vi "Append Report Text (str).vi"(0 "report in":refnum<class "NI_report.lvclass">, 1 "MS Office parameters":T1, 2 "format string (%.3f)":string="%.3f", 7 "text":string, 9 "append on new line? (F)":bool, 11 "error in (no error)":errorcluster) -> (4 "report out":refnum<class "NI_report.lvclass">, 8 "start out (Word)":i32, 10 "end out (Word)":i32, 15 "error out":errorcluster)   [LabVIEW 2020, in "NI_report.lvclass"]
doc: "Appends text to the selected report."
uses:
  <vilib>/Utility/NIReport.llb/NI_report.lvclass
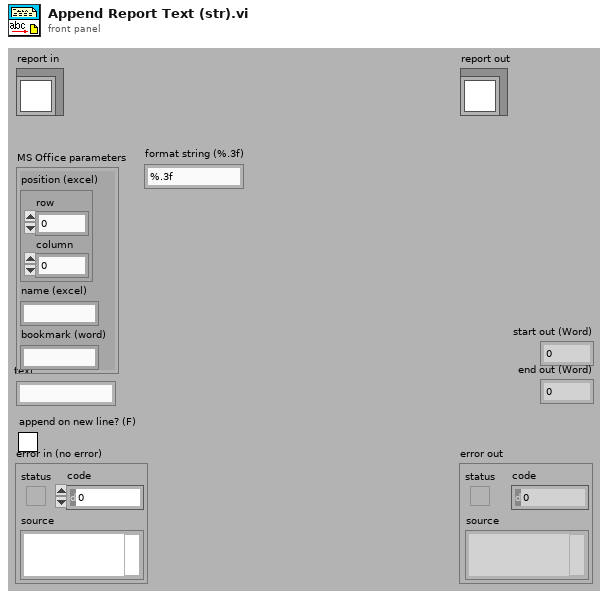
[diagram p1: front panel]
types:
  T1 = cluster{"position (excel)":cluster{"row":i32, "column":i32}, "name (excel)":string, "bookmark (word)":string}
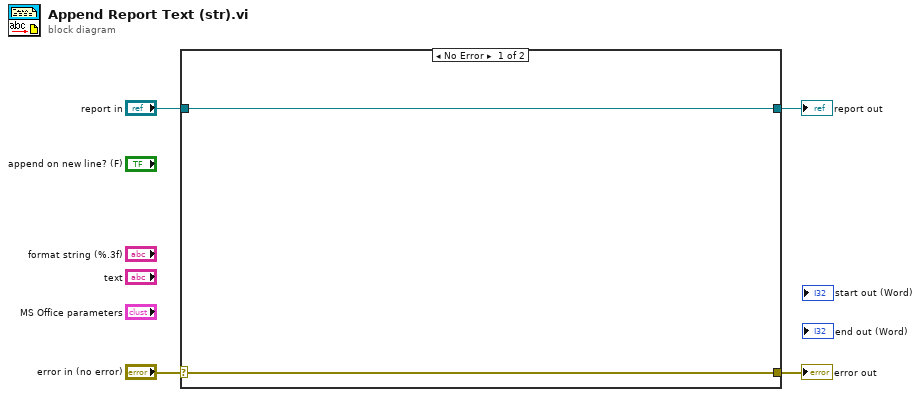
[diagram p0: block diagram]
diagram:
  n1 = case shown="No Error" "error in (no error)" {
    selector: "error in (no error)" -> [w5 w8]
    tunnel: [w5 w8] -> w3
    tunnel: [w6 w7] -> w1
    tunnel: "report in" -> [w6 w7]
    frame No Error {
    }
    frame Error {
    }
  }
  "error out" <- w3
  "report out" <- w1
